vi "PGPASS.UserMgr.vi"(8 "error in (no error)":errorcluster) -> (0 "error out":errorcluster)   [LabVIEW 2019, in "PGPASS.lvlib"]
uses:
  PGPASS.lvlib
  PGPASS.Connection Information.ctl
panel:
  in  "Login":bool
  in  "Users":i32(listbox)
  in  "Exit":bool
  in  "Delete User":bool
  in  "Add User":bool
  in  "Host":string
  in  "Port":string
  in  "Database":string
  in  "Username":string
  in  "Password":string
  # "PGPASS: User Manager"
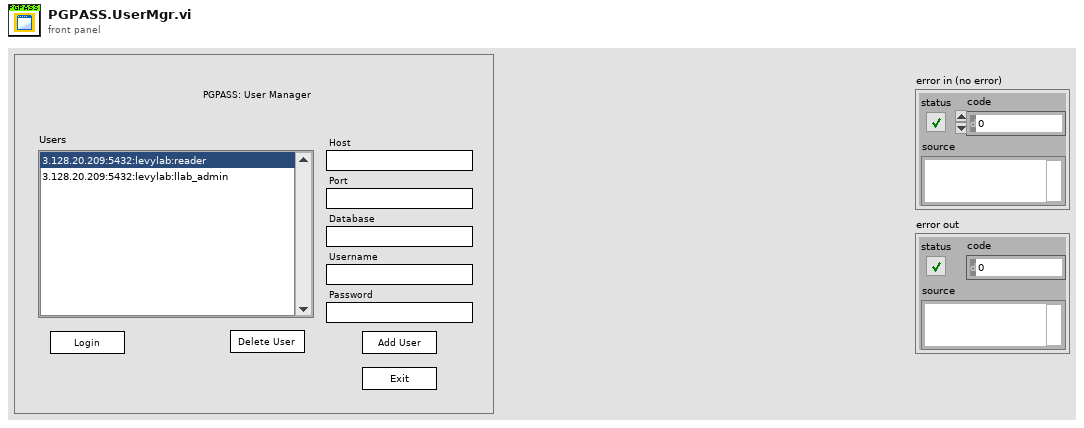
[diagram p1: front panel]
types:
  T1 = typedef "PGPASS.lvlib/PGPASS.Connection Information.ctl" = cluster{"host":string, "port":string, "dbname":string, "user":string, "password":string}
  T2 = enum32{"Invalid", "Standard", "Closed", "Hidden", "Minimized", "Maximized"}
  T3 = enum32{"invalid app kind", "Development System", "Run Time System", "Student Edition", "Embedded LabVIEW", "Evaluation", "Custom"}
  T4 = cluster{"Core":cluster{"Current VI Reference":refnum<vi>, "Close Panel on Exit?":bool}, "Connections":T1[], "New User":T1}
  T5 = cluster{"Current VI Reference":refnum<vi>, "Close Panel on Exit?":bool}
  T6 = cluster{"host":string, "dbname":string, "user":string}
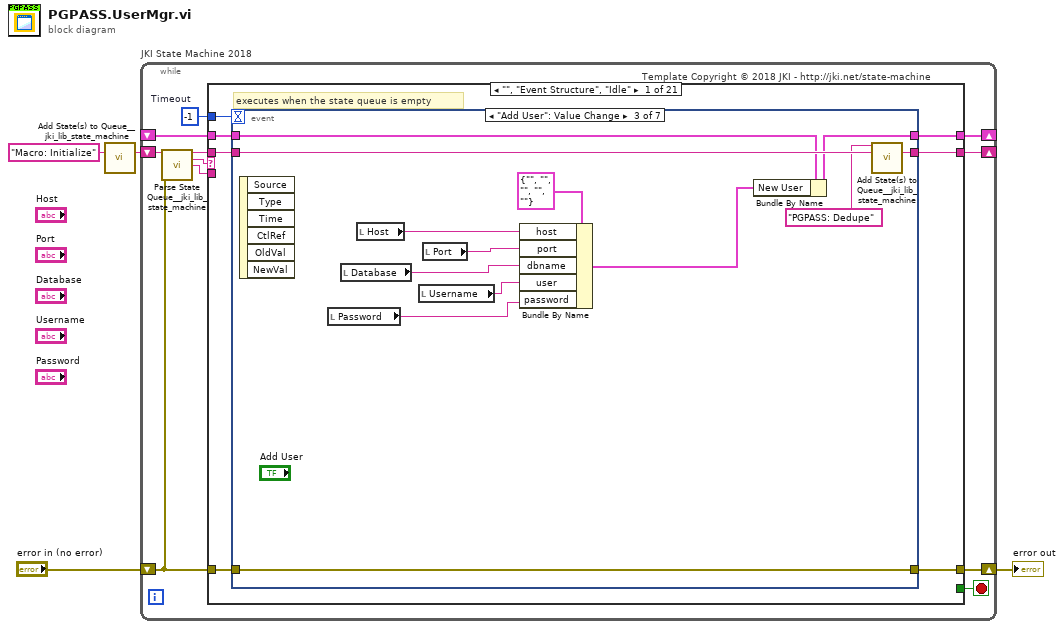
[diagram p0: block diagram]
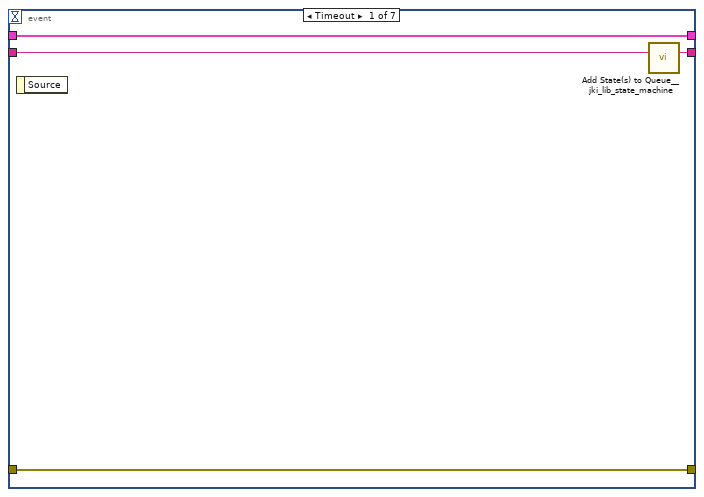
[diagram p2: hidden frame]
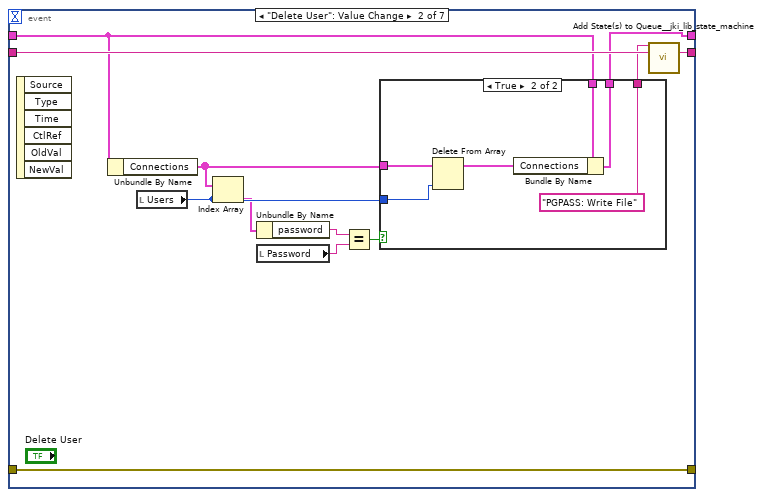
[diagram p3: hidden frame]
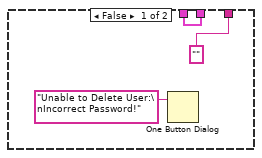
[diagram p4: hidden frame]
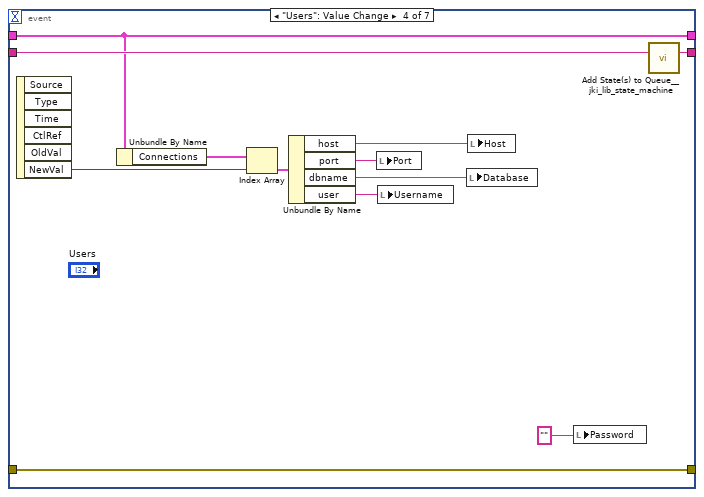
[diagram p5: hidden frame]
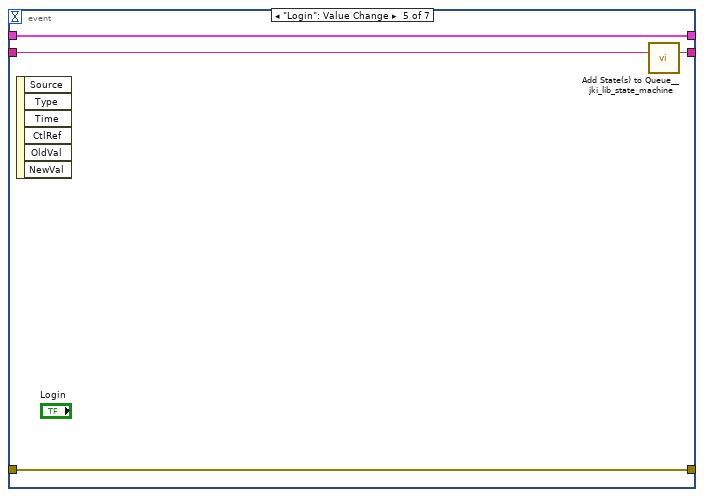
[diagram p6: hidden frame]
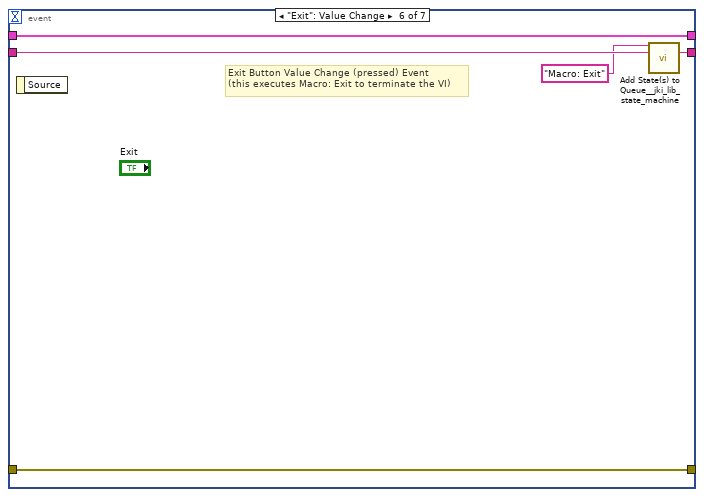
[diagram p7: hidden frame]
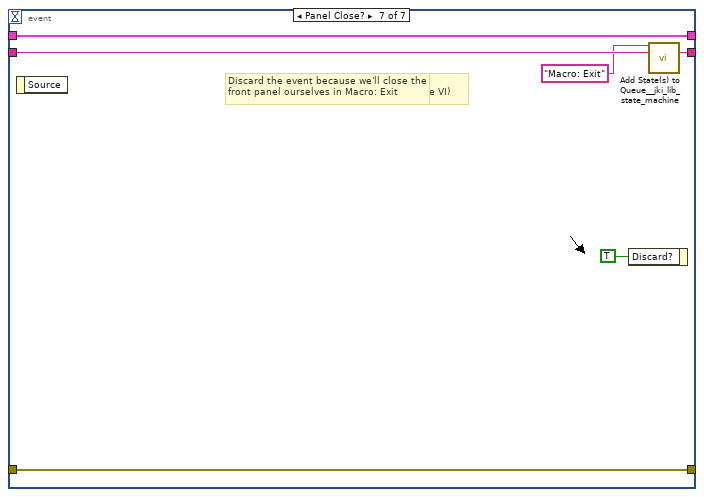
[diagram p8: hidden frame]
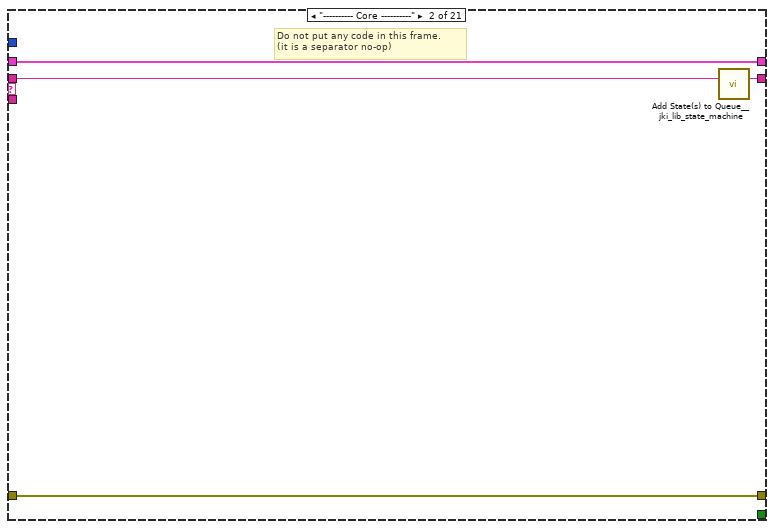
[diagram p9: hidden frame]
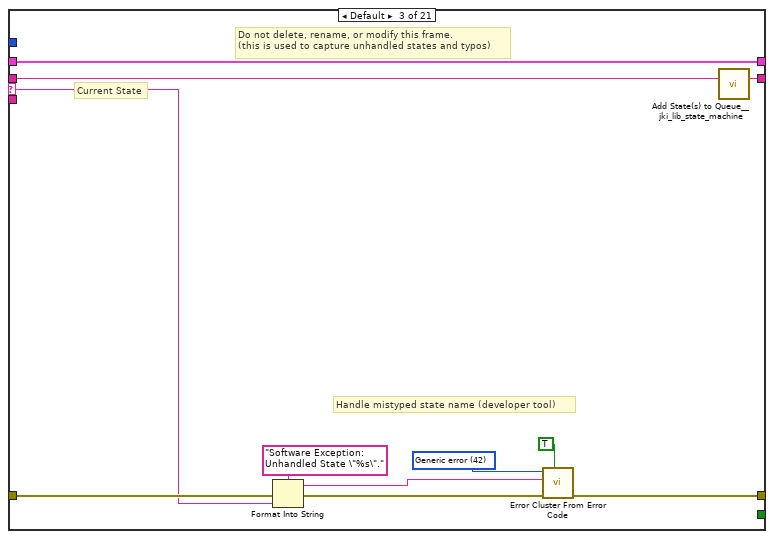
[diagram p10: hidden frame]
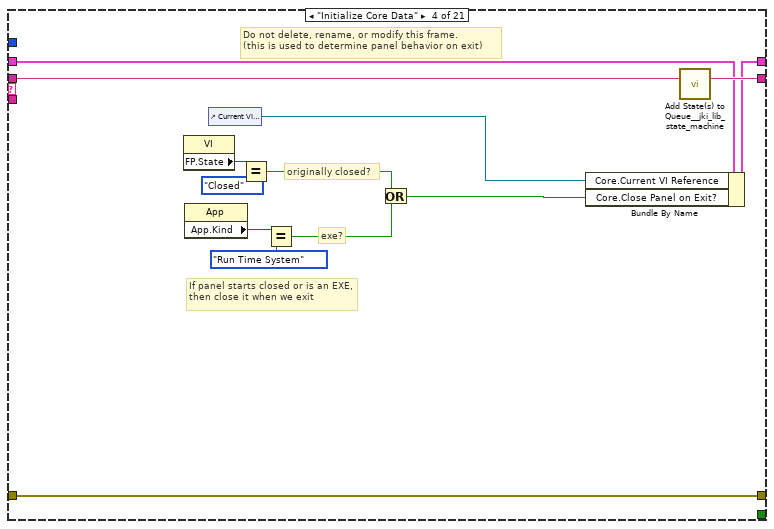
[diagram p11: hidden frame]
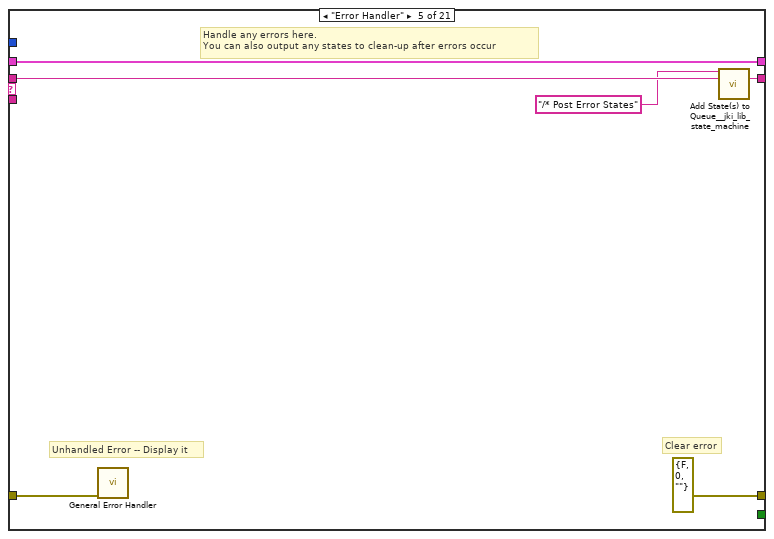
[diagram p12: hidden frame]
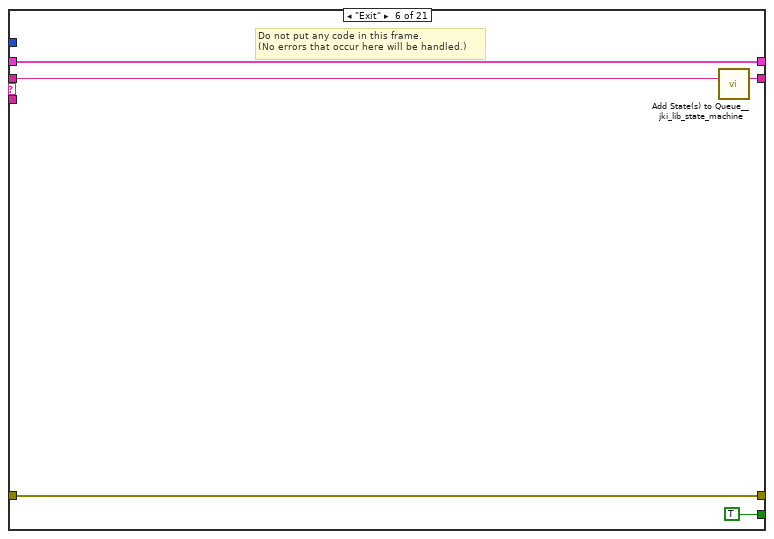
[diagram p13: hidden frame]
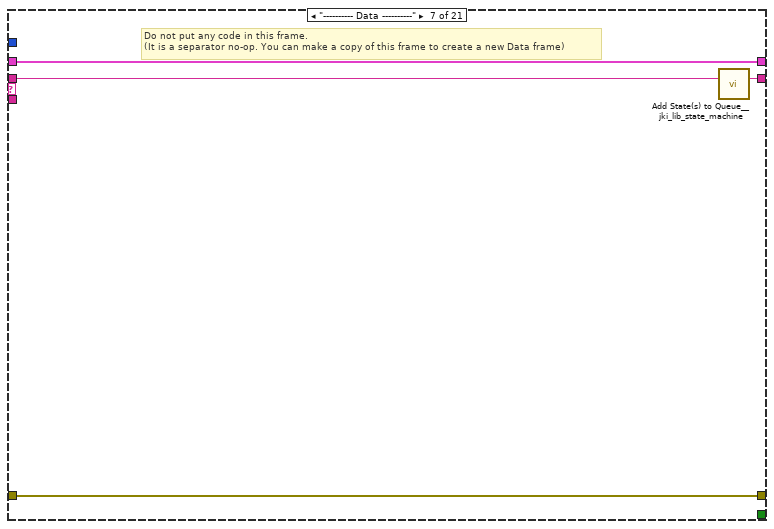
[diagram p14: hidden frame]
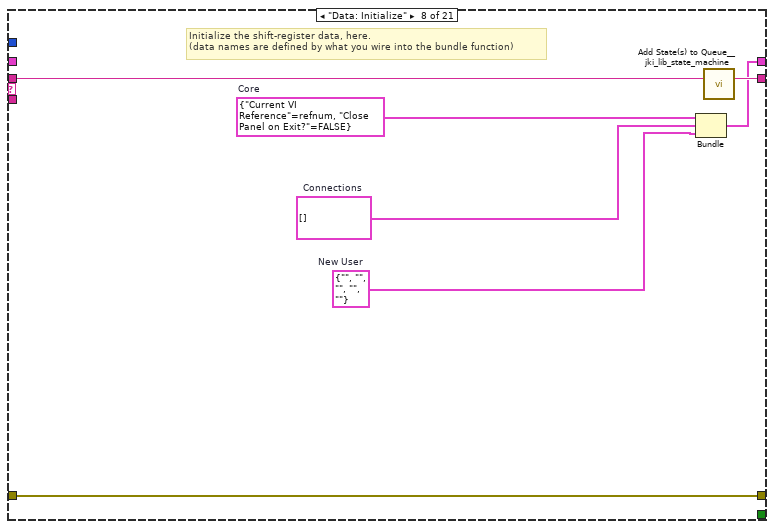
[diagram p15: hidden frame]
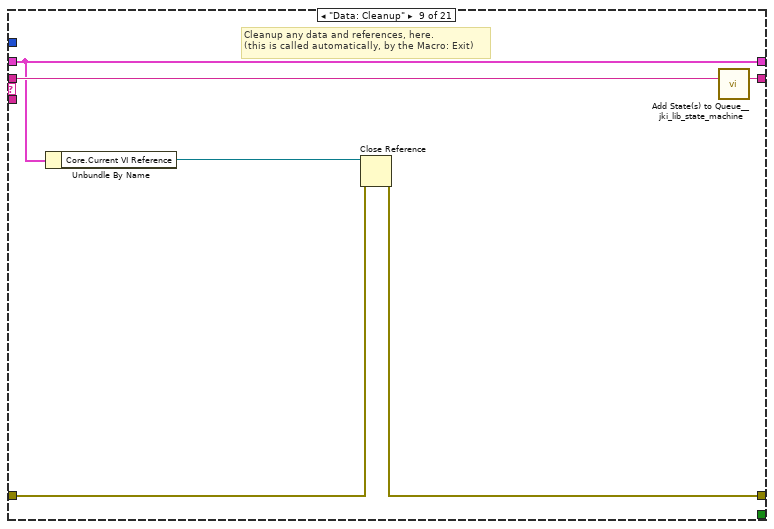
[diagram p16: hidden frame]
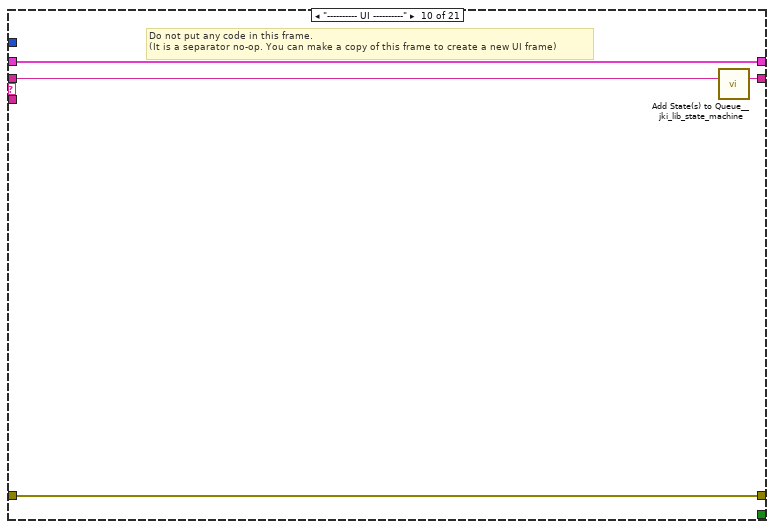
[diagram p17: hidden frame]
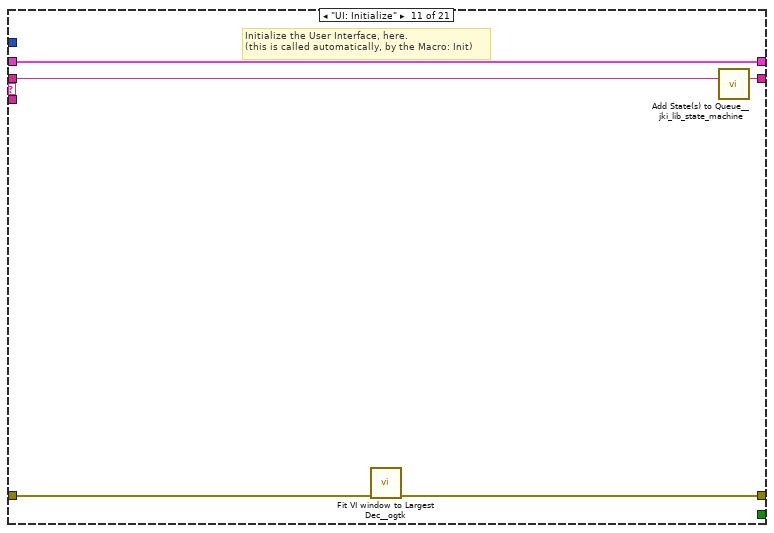
[diagram p18: hidden frame]
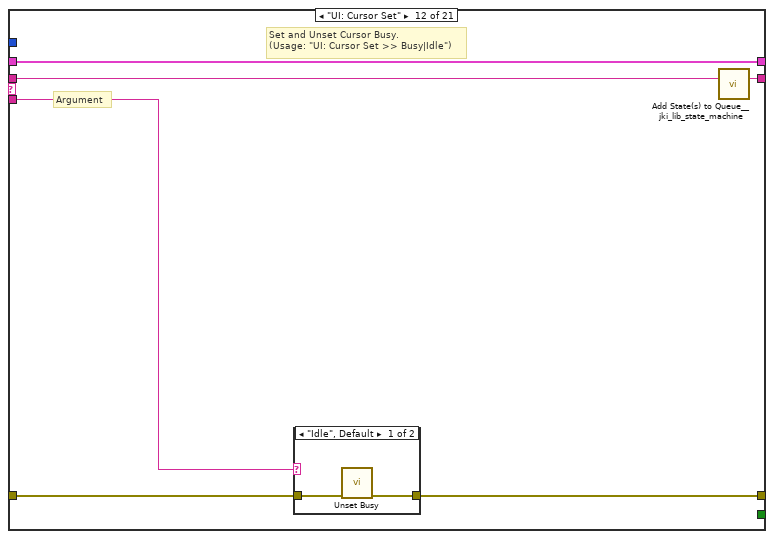
[diagram p19: hidden frame]
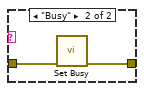
[diagram p20: hidden frame]
diagram:
  n1 = call <vilib>:"Add State(s) to Queue__jki_lib_state_machine.vi"("State(s) in (\"\")"="Macro: Initialize") -> ("States Out"=w4:string)  [unwired: 14 in]
  n2 = while "JKI State Machine 2018" {
    shift-right: [w8] -> _
    shift-left: _ -> [w7]
    shift-right: [w11] -> w2
    shift-left: "error in (no error)" -> [w5]
    shift-right: [w10] -> _
    shift-left: w4 -> [w12]
    stop <- w9 stop-if-true
    w6 = -1  # Timeout
    # "Template Copyright © 2018 JKI - http://jki.net/state-machine"
    n3 = call <vilib>:"Parse State Queue__jki_lib_state_machine.vi"("State Queue"=w12, "Error In (no error)"=w5) -> ("Remaining States"=w14:string, "Current State"=w15:string, "Arguments"=w13:string)  [unwired: 11 in]
    n4 = case shown="\"\", \"Event Structure\", \"Idle\"" w15 {
      selector: w15 -> [_ _ w92 _ _ _ _ _ _ _ _ _ _ _ _ _ _ _ _ _ _]
      tunnel: w14 -> [w22 w91 w96 w115 w121 w126 w130 w137 w143 w147 w152 w158 w169 w241 w252 w257 w267 w271 w279 w286 w302]
      tunnel: w13 -> [_ _ _ _ _ _ _ _ _ _ _ w153 w163 _ _ _ _ _ _ _ _]
      tunnel: w7 -> [w20 w88 w94 w108 w118 w124 w127 _ w138 w144 w150 w156 w165 w237 w249 w254 w264 w268 w273 w284 w290]
      tunnel: [w19 w89 w98 w112 errorcluster {"status"=FALSE, "code"=0, "source"=""} ("error out") w123 w128 w134 w139 w145 w149 w154 w166 w239 w250 w255 w265 w269 w277 w282 w300] -> w11
      tunnel: w5 -> [w18 w89 w97 w112 w117 w123 w128 w134 w140 w145 w148 w155 w167 w239 w250 w255 w265 w269 w276 w283 w300]
      tunnel: [w21 w90 w95 w114 w120 w125 w129 w136 w142 w146 w151 w157 w168 w240 w251 w256 w266 w270 w278 w285 w301] -> w10
      tunnel: [_ _ _ _ _ TRUE _ _ _ _ _ _ _ _ _ _ _ _ _ _ _] -> w9
      tunnel: [w17 w88 w94 w113 w118 w124 w127 w135 w138 w144 w150 w156 w165 w237 w249 w254 w264 w268 w274 w284 w289] -> w8
      tunnel: w6 -> [w16 _ _ _ _ _ _ _ _ _ _ _ _ _ _ _ _ _ _ _ _]
      frame "", "Event Structure", "Idle" {
        # "executes when the state queue is empty"
        n5 = event shown="[2] \"Add User\": Value Change" {
          selector: _ -> [_ _ _ _ _ _ _]
          dyn-events: _ -> [_ _ _ _ _ _ _]
          timeout: w16 -> [_ _ _ _ _ _ _]
          tunnel: w22 -> [w26 w38 w60 w72 w76 w81 w87]
          tunnel: [w25 w37 w59 w71 w75 w80 w86] -> w21
          tunnel: w20 -> [w23 w35 w52 w64 w73 w78 w84]
          tunnel: [w24 w36 w58 w70 w74 w79 w85] -> w19
          tunnel: w18 -> [w24 w36 w58 w70 w74 w79 w85]
          tunnel: [w23 w34 w53 w64 w73 w78 w84] -> w17
          event Timeout {
            n6 = event-data() -> ()  [unwired: 1 in, 1 out]
            n7 = call <vilib>:"Add State(s) to Queue__jki_lib_state_machine.vi"("State(s) in (\"\")"=w26) -> ("States Out"=w25:string)  [unwired: 14 in]
          }
          event "Delete User": Value Change {
            n8 = event-data() -> ()  [unwired: 1 in, 6 out]
            n9 = Unbundle By Name(w35) -> ("Connections"=w33:T1[])
            n10 = local read "Users"() -> (w32:i32)
            n11 = Index Array(array=w33, index=w32) -> (element=w31:T1)
            n12 = Unbundle By Name(w31) -> ("password"=w30:string)
            n13 = local read "Password"() -> (w29:string)
            n14 = Equal?(x=w30, y=w29) -> (x = y?=w28:bool)
            n15 = case shown="True" w28 {
              tunnel: w35 -> [w41 w47]
              tunnel: [w41 w46] -> w34
              tunnel: w33 -> [_ w45]
              tunnel: w32 -> [_ w44]
              tunnel: ["" ("State(s) in Front (\"\")") "PGPASS: Write File" ("State(s) in Front (\"\")")] -> w27
              frame False {
                n16 = One Button Dialog(message="Unable to Delete User:\nIncorrect Password!") -> ()  [unwired: 1 in, 1 out]
              }
              frame True {
                n17 = Delete From Array(array=w45, index=w44) -> (array with subset deleted=w42:T1[])  [unwired: 1 in, 1 out]
                n18 = Bundle By Name(cluster=w47, "Connections"=w42) -> (w46:T4)
              }
            }
            n19 = call <vilib>:"Add State(s) to Queue__jki_lib_state_machine.vi"("State(s) in Front (\"\")"=w27, "State(s) in (\"\")"=w38) -> ("States Out"=w37:string)  [unwired: 13 in]
          }
          event "Add User": Value Change {
            n20 = event-data() -> ()  [unwired: 1 in, 6 out]
            n21 = local read "Password"() -> (w57:string)
            n22 = local read "Database"() -> (w56:string)
            n23 = local read "Host"() -> (w54:string)
            n24 = local read "Username"() -> (w50:string)
            n25 = local read "Port"() -> (w55:string)
            n26 = Bundle By Name(cluster=T1 {"host"="", "port"="", "dbname"="", "user"="", "password"=""} ("input cluster"), "host"=w54, "port"=w55, "dbname"=w56, "user"=w50, "password"=w57) -> (w48:T1)
            n27 = Bundle By Name(cluster=w52, "New User"=w48) -> (w53:T4)
            n28 = call <vilib>:"Add State(s) to Queue__jki_lib_state_machine.vi"("State(s) in Front (\"\")"="PGPASS: Dedupe" ("State(s) in Front (\"\")"), "State(s) in (\"\")"=w60) -> ("States Out"=w59:string)  [unwired: 13 in]
          }
          event "Users": Value Change {
            n29 = event-data() -> ("NewVal"=w65:i32)  [unwired: 1 in, 5 out]
            n30 = Unbundle By Name(w64) -> ("Connections"=w63:T1[])
            n31 = Index Array(array=w63, index=w65) -> (element=w61:T1)
            n32 = Unbundle By Name(w61) -> ("host"=w67:string, "port"=w68:string, "dbname"=w69:string, "user"=w62:string)
            n33 = local write "Port"(w68) -> ()
            n34 = local write "Username"(w62) -> ()
            n35 = local write "Database"(w69) -> ()
            n36 = local write "Host"(w67) -> ()
            n37 = local write "Password"("" ("password")) -> ()
            n38 = call <vilib>:"Add State(s) to Queue__jki_lib_state_machine.vi"("State(s) in (\"\")"=w72) -> ("States Out"=w71:string)  [unwired: 14 in]
          }
          event "Login": Value Change {
            n39 = event-data() -> ()  [unwired: 1 in, 6 out]
            n40 = call <vilib>:"Add State(s) to Queue__jki_lib_state_machine.vi"("State(s) in (\"\")"=w76) -> ("States Out"=w75:string)  [unwired: 14 in]
          }
          event "Exit": Value Change {
            # "Exit Button Value Change (pressed) Event\n(this executes Macro: Exit to terminate the VI)"
            n41 = event-data() -> ()  [unwired: 1 in, 1 out]
            n42 = call <vilib>:"Add State(s) to Queue__jki_lib_state_machine.vi"("State(s) in Front (\"\")"="Macro: Exit", "State(s) in (\"\")"=w81) -> ("States Out"=w80:string)  [unwired: 13 in]
          }
          event Panel Close? {
            # "Discard the event because we'll close the front panel ourselves in Macro: Exit"
            # "Close Panel button (pressed) Event\n(this executes Macro: Exit to terminate the VI)"
            n43 = event-data() -> ()  [unwired: 1 in, 1 out]
            n44 = event-data("Discard?"=TRUE) -> ()  [unwired: 1 in, 1 out]
            n45 = call <vilib>:"Add State(s) to Queue__jki_lib_state_machine.vi"("State(s) in Front (\"\")"="Macro: Exit", "State(s) in (\"\")"=w87) -> ("States Out"=w86:string)  [unwired: 13 in]
          }
        }
      }
      frame "---------- Core ----------" {
        # "Do not put any code in this frame.\n(it is a separator no-op)"
        n46 = call <vilib>:"Add State(s) to Queue__jki_lib_state_machine.vi"("State(s) in (\"\")"=w91) -> ("States Out"=w90:string)  [unwired: 14 in]
      }
      frame Default {
        w101 = 42 items=["No error", "Argument error", "Memory is full", "Out of zone", "End of file", "File already open", "Generic file I/O error", "File not found", "File permission error", "Disk is full", "Duplicate path", "Too many files open", "System feature not enabled", "Resource file not found", "Cannot add resource", "Resource not found", "Image not found", "Image memory error", "Pen does not exist", "Config type invalid", "Config token not found", "Config parse error", "Config memory error", "Bad external code format", "Bad external code offset", "External code not present", "Null window", "Destroy window error", "Null menu", "Print aborted", "Bad print record", "Print driver error", "Windows error during printing", "Memory error during printing", "Print dialog error", "Generic print error", "Invalid device refnum", "Device not found", "Device parameter error", "Device unit error", "Cannot open device", "Device call aborted", "Generic error", "Cancelled by user", "Object ID too low", "Object ID too high", "Object not in heap", "Unknown heap", "Unknown object (invalid DefProc)", "Unknown object (DefProc not in table)", "Message out of range", "Invalid (null) method", "Unknown message", "Manager call not supported", "Bad address", "Network operation in progress", "Network operation timed out", "Connection is busy", "Network attribute not supported", "Network error", "Address in use", "System out of memory", "Connection aborted", "Connection refused", "Not connected", "Already connected", "Connection closed", "Initialization error (interapplication manager)", "Bad occurrence", "Wait on unbound occurrence handler", "Occurrence queue overflow", "Datalog type conflict", "Unused", "Unrecognized type (interapplication manager)", "Memory corrupt", "Failed to make temporary DLL", "Old CIN version", "Drag socket not found", "Failed to load drop-object", "Failed to register OLE object", "Failed to release OLE object", "Format specifier type mismatch", "Unknown format specifier", "Too few format specifiers", "Too many format specifiers", "Scan failed", "Newer CIN version", "Error converting to variant", "Runtime menu error", "Password tampered", "Variant attribute not found", "Incompatible variant data type", "Event data is not available", "Event Store is not present", "Occurrence is not found", "Event Queue is not created", "Event info is not available", "Refnum passed is NULL", "Error retrieving Class GUID", "Error retrieving CoClass GUID", "Error retrieving TypeLib GUID.", "Bad built application magic bytes.", "Specific driver is different from the specific driver associated with the Logical Name.", "There is no session opened to the class driver.", "Max Error", "MAX - Error with config objects", "MAX - Error loading configuration", "MAX - Group not supported"]
        # "Current State"
        # "Do not delete, rename, or modify this frame.\n(this is used to capture unhandled states and typos)"
        # "Handle mistyped state name (developer tool)"
        n47 = Format Into String(format string="Software Exception: Unhandled State \"%s\"." ("message"), error in=w97, w92) -> (resulting string=w100:string, error out=w99:errorcluster)  [unwired: 1 in]
        n48 = call <vilib>:"Error Cluster From Error Code.vi"("show call chain? (False)"=TRUE, "error in (no error)"=w99, "error message (\"\")"=w100, "error code (0)"=w101) -> ("error out"=w98:errorcluster)  [unwired: 5 in]
        n49 = call <vilib>:"Add State(s) to Queue__jki_lib_state_machine.vi"("State(s) in (\"\")"=w96) -> ("States Out"=w95:string)  [unwired: 14 in]
      }
      frame "Initialize Core Data" {
        # "Do not delete, rename, or modify this frame.\n(this is used to determine panel behavior on exit)"
        # "originally closed?"
        # "exe?"
        # "If panel starts closed or is an EXE, then close it when we exit"
        n50 = property class="VI"() -> ("FP.State"=w105:T2)  [unwired: 2 in, 2 out]
        n51 = property class="App"() -> ("App.Kind"=w111:T3)  [unwired: 2 in, 2 out]
        n52 = control-ref of="Current VI Reference"() -> (w106:refnum<vi>)
        n53 = Equal?(x=w105, y=T2."Closed" ("Front Panel Window:State")) -> (x = y?=w103:bool)
        n54 = Equal?(x=w111, y=T3."Run Time System" ("Application:Kind")) -> (x = y?=w109:bool)
        n55 = Or(x=w103, y=w109) -> (x .or. y?=w107:bool)
        n56 = Bundle By Name(cluster=w108, "Core.Current VI Reference"=w106, "Core.Close Panel on Exit?"=w107) -> (w113:T4)
        n57 = call <vilib>:"Add State(s) to Queue__jki_lib_state_machine.vi"("State(s) in (\"\")"=w115) -> ("States Out"=w114:string)  [unwired: 14 in]
      }
      frame "Error Handler" {
        # "Unhandled Error -- Display it"
        # "Handle any errors here.\nYou can also output any states to clean-up after errors occur"
        # "Clear error"
        n58 = call <vilib>:"General Error Handler.vi"("error in (no error)"=w117) -> ()  [unwired: 10 in, 5 out]
        n59 = call <vilib>:"Add State(s) to Queue__jki_lib_state_machine.vi"("State(s) in Front (\"\")"="/* Post Error States", "State(s) in (\"\")"=w121) -> ("States Out"=w120:string)  [unwired: 13 in]
      }
      frame "Exit" {
        # "Do not put any code in this frame.\n(No errors that occur here will be handled.)"
        n60 = call <vilib>:"Add State(s) to Queue__jki_lib_state_machine.vi"("State(s) in (\"\")"=w126) -> ("States Out"=w125:string)  [unwired: 14 in]
      }
      frame "---------- Data ----------" {
        # "Do not put any code in this frame.\n(It is a separator no-op. You can make a copy of this frame to create a new Data frame)"
        n61 = call <vilib>:"Add State(s) to Queue__jki_lib_state_machine.vi"("State(s) in (\"\")"=w130) -> ("States Out"=w129:string)  [unwired: 14 in]
      }
      frame "Data: Initialize" {
        w131 = T1 {"host"="", "port"="", "dbname"="", "user"="", "password"=""}  # New User
        w132 = T1[] []  # Connections
        w133 = T5 {"Current VI Reference"=refnum, "Close Panel on Exit?"=FALSE}  # Core
        # "Initialize the shift-register data, here.\n(data names are defined by what you wire into the bundle function)"
        n62 = Bundle("Core"=w133, "Connections"=w132, "New User"=w131) -> (w135:T4)  [unwired: 1 in]
        n63 = call <vilib>:"Add State(s) to Queue__jki_lib_state_machine.vi"("State(s) in (\"\")"=w137) -> ("States Out"=w136:string)  [unwired: 14 in]
      }
      frame "Data: Cleanup" {
        # "Cleanup any data and references, here.\n(this is called automatically, by the Macro: Exit)"
        n64 = Unbundle By Name(w138) -> ("Core.Current VI Reference"=w141:refnum<vi>)
        n65 = Close Reference(reference=w141, error in (no error)=w140) -> (error out=w139:errorcluster)
        n66 = call <vilib>:"Add State(s) to Queue__jki_lib_state_machine.vi"("State(s) in (\"\")"=w143) -> ("States Out"=w142:string)  [unwired: 14 in]
      }
      frame "---------- UI ----------" {
        # "Do not put any code in this frame.\n(It is a separator no-op. You can make a copy of this frame to create a new UI frame)"
        n67 = call <vilib>:"Add State(s) to Queue__jki_lib_state_machine.vi"("State(s) in (\"\")"=w147) -> ("States Out"=w146:string)  [unwired: 14 in]
      }
      frame "UI: Initialize" {
        # "Initialize the User Interface, here.\n(this is called automatically, by the Macro: Init)"
        n68 = call <userlib>:"Fit VI window to Largest Dec__ogtk.vi"("error in (no error)"=w148) -> ("error out"=w149:errorcluster)  [unwired: 5 in, 1 out]
        n69 = call <vilib>:"Add State(s) to Queue__jki_lib_state_machine.vi"("State(s) in (\"\")"=w152) -> ("States Out"=w151:string)  [unwired: 14 in]
      }
      frame "UI: Cursor Set" {
        # "Argument"
        # "Set and Unset Cursor Busy.\n(Usage: \"UI: Cursor Set >> Busy|Idle\")"
        n70 = case shown="\"Idle\", Default" w153 {
          tunnel: w155 -> [w160 w162]
          tunnel: [w159 w161] -> w154
          frame "Idle", Default {
            n71 = call <vilib>:"Unset Busy.vi"("error in (no error)"=w160) -> ("error out"=w159:errorcluster)  [unwired: 10 in]
          }
          frame "Busy" {
            n72 = call <vilib>:"Set Busy.vi"("error in (no error)"=w162) -> ("error out"=w161:errorcluster)  [unwired: 9 in, 1 out]
          }
        }
        n73 = call <vilib>:"Add State(s) to Queue__jki_lib_state_machine.vi"("State(s) in (\"\")"=w158) -> ("States Out"=w157:string)  [unwired: 14 in]
      }
      frame "UI: Front Panel State" {
        # "Argument"
        # "Set Front Panel Open or Closed\n(Usage: \"UI: Front Panel State >> Open|Close\")"
        n74 = Unbundle By Name(w165) -> ("Core.Current VI Reference"=w164:refnum<vi>)
        n75 = case shown="\"Minimize\", \"Minimized\"" w163 {
          tunnel: w167 -> [w175 w190 w201 w214 w227]
          tunnel: [w177 w191 w203 w216 w229] -> w166
          tunnel: w164 -> [w176 w188 w202 w215 w228]
          frame "Open", "Standard", Default {
            w170 = T2."Standard" ("State")
            n76 = property class="VI"(reference=w176, error in=w175) -> (reference out=w173:refnum<vi>, error out=w174:errorcluster, "FP.State"=w172:T2)
            n77 = Not Equal?(x=w172, y=w170) -> (x != y?=w171:bool)
            n78 = case shown="True" w171 {
              tunnel: [w181 w183] -> w177
              tunnel: w174 -> [w180 w183]
              tunnel: w173 -> [w179 _]
              tunnel: w170 -> [w178 _]
              frame True {
                n79 = invoke class="VI" method="FP.Open"(reference=w179, error in=w180, "Activate"=TRUE, "State"=w178) -> (error out=w181:errorcluster)  [unwired: 1 in, 4 out]
              }
              frame False {
              }
            }
          }
          frame "Close", "Closed" {
            n80 = property class="VI"(reference=w188, error in=w190) -> (reference out=w187:refnum<vi>, error out=w189:errorcluster, "FP.State"=w185:T2)
            n81 = Not Equal?(x=w185, y=T2."Closed" ("Front Panel Window:State")) -> (x != y?=w184:bool)
            n82 = case shown="True" w184 {
              tunnel: [w192 w195] -> w191
              tunnel: w189 -> [w192 w194]
              tunnel: w187 -> [_ w193]
              frame False {
              }
              frame True {
                n83 = invoke class="VI" method="FP.Close"(reference=w193, error in=w194) -> (error out=w195:errorcluster)  [unwired: 1 in, 2 out]
              }
            }
          }
          frame "Hidden", "Hide" {
            w196 = T2."Hidden" ("State")
            n84 = property class="VI"(reference=w202, error in=w201) -> (reference out=w199:refnum<vi>, error out=w200:errorcluster, "FP.State"=w198:T2)
            n85 = Not Equal?(x=w198, y=w196) -> (x != y?=w197:bool)
            n86 = case shown="True" w197 {
              tunnel: [w207 w208] -> w203
              tunnel: w200 -> [w206 w208]
              tunnel: w199 -> [w205 _]
              tunnel: w196 -> [w204 _]
              frame True {
                n87 = invoke class="VI" method="FP.Open"(reference=w205, error in=w206, "State"=w204) -> (error out=w207:errorcluster)  [unwired: 2 in, 4 out]
              }
              frame False {
              }
            }
          }
          frame "Minimize", "Minimized" {
            w209 = T2."Minimized" ("State")
            n88 = property class="VI"(reference=w215, error in=w214) -> (reference out=w212:refnum<vi>, error out=w213:errorcluster, "FP.State"=w211:T2)
            n89 = Not Equal?(x=w211, y=w209) -> (x != y?=w210:bool)
            n90 = case shown="True" w210 {
              tunnel: [w220 w221] -> w216
              tunnel: w213 -> [w219 w221]
              tunnel: w212 -> [w218 _]
              tunnel: w209 -> [w217 _]
              frame True {
                n91 = invoke class="VI" method="FP.Open"(reference=w218, error in=w219, "State"=w217) -> (error out=w220:errorcluster)  [unwired: 2 in, 4 out]
              }
              frame False {
              }
            }
          }
          frame "Maximize", "Maximized" {
            w222 = T2."Maximized" ("State")
            n92 = property class="VI"(reference=w228, error in=w227) -> (reference out=w225:refnum<vi>, error out=w226:errorcluster, "FP.State"=w224:T2)
            n93 = Not Equal?(x=w224, y=w222) -> (x != y?=w223:bool)
            n94 = case shown="True" w223 {
              tunnel: [w233 w234] -> w229
              tunnel: w226 -> [w232 w234]
              tunnel: w225 -> [w231 _]
              tunnel: w222 -> [w230 _]
              frame True {
                n95 = invoke class="VI" method="FP.Open"(reference=w231, error in=w232, "State"=w230) -> (error out=w233:errorcluster)  [unwired: 2 in, 4 out]
              }
              frame False {
              }
            }
          }
        }
        n96 = call <vilib>:"Add State(s) to Queue__jki_lib_state_machine.vi"("State(s) in (\"\")"=w169) -> ("States Out"=w168:string)  [unwired: 14 in]
      }
      frame "UI: Update User List" {
        # "Do not put any code in this frame.\n(It is a separator no-op. You can make a copy of this frame to create a new UI frame)"
        n97 = Unbundle By Name(w237) -> ("Connections"=w236:T1[])
        n98 = for {
          tunnel: w236 -> [w248] mode=indexing
          tunnel: [w242] -> w238 mode=indexing
          n99 = Unbundle By Name(w248) -> ("host"=w246:string, "port"=w245:string, "dbname"=w244:string, "user"=w243:string)
          n100 = Format Into String(format string="%s:%s:%s:%s", w246, w245, w244, w243) -> (resulting string=w242:string)  [unwired: 2 in, 1 out]
        }
        n101 = property on="Users" class="LstBox (strict)"("Item Names"=w238) -> ()  [unwired: 2 in, 2 out]
        n102 = local write "Password"("" ("Password")) -> ()
        n103 = call <vilib>:"Add State(s) to Queue__jki_lib_state_machine.vi"("State(s) in (\"\")"=w241) -> ("States Out"=w240:string)  [unwired: 14 in]
      }
      frame "---------- Macro ----------" {
        # "Do not put any code in this frame.\n(It is a separator no-op. You can make a copy of this frame to create a new Macro frame)"
        n104 = call <vilib>:"Add State(s) to Queue__jki_lib_state_machine.vi"("State(s) in (\"\")"=w252) -> ("States Out"=w251:string)  [unwired: 14 in]
      }
      frame "Macro: Initialize" {
        w253 = "Data: Initialize\nInitialize Core Data\nUI: Initialize\nUI: Front Panel State >> Open\n\nPGPASS: Read File"  # Data: Initialize Initialize Core Data UI: Initialize UI: Front Panel State >> Open  PGPASS: Read File
        # "Initialization Macro\n(This is called once, when the VI starts)"
        n105 = call <vilib>:"Add State(s) to Queue__jki_lib_state_machine.vi"("State(s) in Front (\"\")"=w253, "State(s) in (\"\")"=w257) -> ("States Out"=w256:string)  [unwired: 13 in]
      }
      frame "Macro: Exit" {
        # "Exit Macro\n(This is called once, when the VI exits)"
        n106 = Unbundle By Name(w264) -> ("Core.Close Panel on Exit?"=w263:bool)
        n107 = Select(t="UI: Front Panel State >> Close", s=w263, f="") -> (s? t:f=w260:string)
        n108 = call <vilib>:"Add State(s) to Queue__jki_lib_state_machine.vi"("State(s) in (\"\")"=w260, "State(s) at Back (\"\")"="Data: Cleanup\nExit") -> ("States Out"=w258:string)  [unwired: 13 in]
        n109 = call <vilib>:"Add State(s) to Queue__jki_lib_state_machine.vi"("State(s) in Front (\"\")"=w258, "State(s) in (\"\")"=w267) -> ("States Out"=w266:string)  [unwired: 13 in]
      }
      frame "---------- PGPASS ----------" {
        # "Template Separator\n(You can make a copy of, or modify, this frame)"
        n110 = call <vilib>:"Add State(s) to Queue__jki_lib_state_machine.vi"("State(s) in (\"\")"=w271) -> ("States Out"=w270:string)  [unwired: 14 in]
      }
      frame "PGPASS: Read File" {
        # "Read PGPASS file\n(and populate Connections array)"
        n111 = call "PGPASS.Read.vi"("error in"=w276) -> ("error out"=w277:errorcluster, "Connections"=w275:T1[])  [unwired: 9 in]
        n112 = Bundle By Name(cluster=w273, "Connections"=w275) -> (w274:T4)
        n113 = call <vilib>:"Add State(s) to Queue__jki_lib_state_machine.vi"("State(s) in Front (\"\")"="UI: Update User List" ("State(s) in Front (\"\")"), "State(s) in (\"\")"=w279) -> ("States Out"=w278:string)  [unwired: 13 in]
      }
      frame "PGPASS: Write File" {
        # "Read PGPASS file\n(and populate Connections array)"
        n114 = Unbundle By Name(w284) -> ("Connections"=w281:T1[])
        n115 = call "PGPASS.Write.vi"("error in"=w283, "Connections"=w281) -> ("error out"=w282:errorcluster)  [unwired: 9 in]
        n116 = call <vilib>:"Add State(s) to Queue__jki_lib_state_machine.vi"("State(s) in Front (\"\")"="UI: Update User List" ("State(s) in Front (\"\")"), "State(s) in (\"\")"=w286) -> ("States Out"=w285:string)  [unwired: 13 in]
      }
      frame "PGPASS: Dedupe" {
        # "Read PGPASS file\n(and populate Connections array)"
        n117 = Unbundle By Name(w290) -> ("Connections"=w292:T1[], "New User"=w291:T1)
        n118 = for {
          tunnel: w292 -> [w314] mode=indexing
          tunnel: [w310] -> w296 mode=indexing
          n119 = Unbundle By Name(w314) -> ("host"=w313:string, "dbname"=w312:string, "user"=w311:string)
          n120 = Bundle("host"=w313, "dbname"=w312, "user"=w311) -> (w310:T6)  [unwired: 1 in]
        }
        n121 = Unbundle By Name(w291) -> ("host"=w299:string, "dbname"=w298:string, "user"=w297:string)
        n122 = Bundle("host"=w299, "dbname"=w298, "user"=w297) -> (w295:T6)  [unwired: 1 in]
        n123 = Search 1D Array(1D array=w296, element=w295) -> (index of element=w294:i32)  [unwired: 1 in]
        n124 = Greater Or Equal To 0?(x=w294) -> (x >= 0?=w293:bool)
        n125 = case shown="False" w293 {
          tunnel: w292 -> [w306 w307]
          tunnel: w291 -> [w305 _]
          tunnel: ["PGPASS: Write File" ("State(s) in Front (\"\")") "" ("State(s) in Front (\"\")")] -> w288
          tunnel: [w303 w307] -> w287
          frame False {
            n126 = Build Array (concatenate)(w306, w305) -> (w303:T1[])
          }
          frame True {
            n127 = One Button Dialog(message="Unable to Add User:\nDuplicate entry!") -> ()  [unwired: 1 in, 1 out]
          }
        }
        n128 = Bundle By Name(cluster=w290, "Connections"=w287) -> (w289:T4)
        n129 = call <vilib>:"Add State(s) to Queue__jki_lib_state_machine.vi"("State(s) in Front (\"\")"=w288, "State(s) in (\"\")"=w302) -> ("States Out"=w301:string)  [unwired: 13 in]
      }
    }
  }
  "error out" <- w2
